vi "AlliGator Load mat FLI Dataset Information.vi"(8 "Error In":errorcluster, 9 "Laser Period":dbl[unit]=5.0000000000000004e-08, 11 "File Path":path) -> (0 "error out":errorcluster, 2 "Metadata":string, 3 "FLI Data File Information":T1, 4 "elapsed (relative) seconds":dbl)   [LabVIEW 2021, in "AlliGator Files.lvlib"]
doc: "Loads HDF5 FLI dataset information."
uses:
  AlliGator Files.lvlib
  HDF5/AlliGator FLI Data File Information.ctl
  Phasor/Phasor Fluorescence Lifetime Parameters v3.ctl
  AlliGator FLI Dataset Type.ctl
  AlliGator SS2 mat FLI File Loading Information.ctl
  AlliGator Load Single Gate Image from SS2 mat File.vi
  <vilib>/addons/h5labview2/base/lib_path.vi
  <vilib>/addons/h5labview2/base/H5Equery.vi
  <vilib>/addons/h5labview2/base/hid_t.ctl
  <vilib>/addons/h5labview2/dataset/H5Dread.llb/H5Dread.xnode
  <vilib>/addons/h5labview2/file/H5F.lvlib
  <vilib>/addons/h5labview2/group/H5G.lvlib
  Time/Time.lvlib
  HDF5/AlliGator HDF5.lvlib
  Phasor/Phasor.lvlib
panel:
  # "see the AlliGator License on the block diagram (Ctrl+E or Window:Show Block Diagram)"
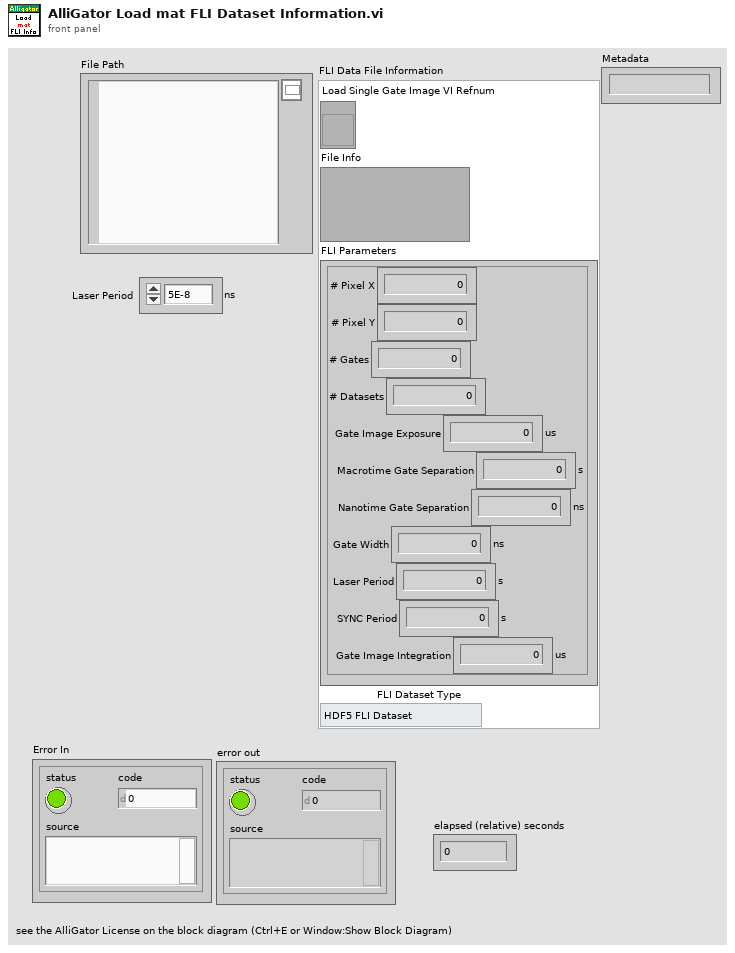
[diagram p1: front panel]
types:
  T1 = typedef "AlliGator HDF5.lvlib/AlliGator FLI Data File Information.ctl" = cluster{"Load Single Gate Image VI Refnum":refnum<vi>, "File Info":variant, "FLI Parameters":T2, "FLI Dataset Type":T3}
  T2 = typedef "Phasor.lvlib/Phasor Fluorescence Lifetime Parameters v3.ctl" = cluster{"# Pixel X":i32, "# Pixel Y":i32, "# Gates":i32, "# Datasets":i32, "Gate Image Exposure":dbl[unit], "Macrotime Gate Separation":dbl[unit], "Nanotime Gate Separation":dbl[unit], "Gate Width":dbl[unit], "Laser Period":dbl[unit], "SYNC Period":dbl[unit], "Gate Image Integration":dbl[unit]}
  T3 = typedef "AlliGator Files.lvlib/AlliGator FLI Dataset Type.ctl" = enum16{"HDF5 FLI Dataset", "Gate Image Folder", ".sdt FLI Dataset (Becker & Hickl)", ".ptu FLI Dataset (PicoQuant)", "SS1 FLI Dataset", "SS2 FLI Dataset", "I/m/phi Dataset", ".bin FLI Dataset (PicoQuant Binned)", ".bin FLI Dataset (Piccolo Binned)", ".mat FLI Dataset"}
  T4 = typedef "AlliGator Files.lvlib/AlliGator SS2 mat FLI File Loading Information.ctl" = cluster{"mat File Path":path, "# Datasets":i32, "# Gates/Dataset":i32}
  T5 = typedef "hid_t.ctl" = i64
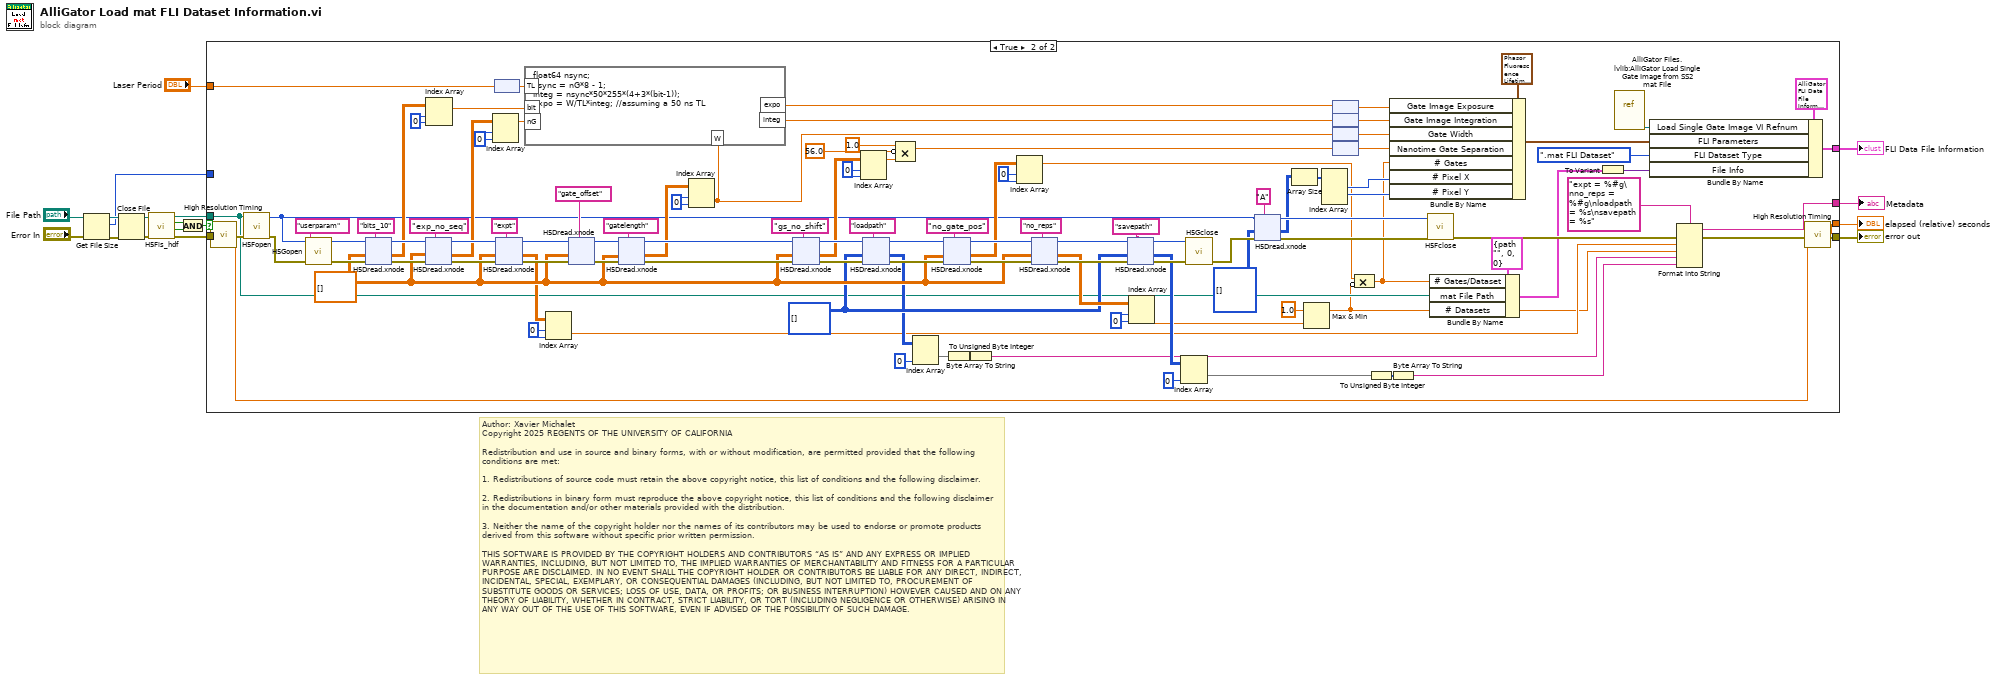
[diagram p0: block diagram]
diagram:
  # "Author: Xavier Michalet\nCopyright 2025 REGENTS OF THE UNIVERSITY OF CALIFORNIA\n\nRedistribution and use in source and binary forms, with or without modification, are permitted provided that the following conditions are met:\n\n1. Redistributions of source code must retain the above copyright notice, this list of conditions and the following disclaimer.\n\n2. Redistributions in binary form must reproduce the above copyright notice, this list of conditions and the following disclaimer in the documentation and/or other materials provided with the distribution.\n\n3. Neither the name of the copyright holder nor the names of its contributors may be used to endorse or promote products derived from this software without specific prior written permission.\n\nTHIS SOFTWARE IS PROVIDED BY THE COPYRIGHT HOLDERS AND CONTRIBUTORS “AS IS” AND ANY EXPRESS OR IMPLIED WARRANTIES, INCLUDING, BUT NOT LIMITED TO, THE IMPLIED WARRANTIES OF MERCHANTABILITY AND FITNESS FOR A PARTICULAR PURPOSE ARE DISCLAIMED. IN NO EVENT SHALL THE COPYRIGHT HOLDER OR CONTRIBUTORS BE LIABLE FOR ANY DIRECT, INDIRECT, INCIDENTAL, SPECIAL, EXEMPLARY, OR CONSEQUENTIAL DAMAGES (INCLUDING, BUT NOT LIMITED TO, PROCUREMENT OF SUBSTITUTE GOODS OR SERVICES; LOSS OF USE, DATA, OR PROFITS; OR BUSINESS INTERRUPTION) HOWEVER CAUSED AND ON ANY THEORY OF LIABILITY, WHETHER IN CONTRACT, STRICT LIABILITY, OR TORT (INCLUDING NEGLIGENCE OR OTHERWISE) ARISING IN ANY WAY OUT OF THE USE OF THIS SOFTWARE, EVEN IF ADVISED OF THE POSSIBILITY OF SUCH DAMAGE."
  n1 = Get File Size(file="File Path", error in="Error In") -> (refnum out=w8:refnum<file>, size (in bytes)=w3:i64, 0:w9:errorcluster)
  n2 = Close File(refnum=w8, error in=w9) -> (path=w7:path, error out=w6:errorcluster)
  n3 = call <vilib>:"H5Fis_hdf.vi"("error in (no error)"=w6, "path in"=w7) -> ("error out"=w13:errorcluster, "valid?"=w16:bool, "exists?"=w17:bool, "path out"=w14:path)  [unwired: 6 in]
  n4 = And(x=w17, y=w16) -> (x .and. y?=w15:bool)
  n5 = case shown="True" w15 {
    tunnel: w14 -> [_ w42]
    tunnel: w13 -> [w18 w128]
    tunnel: [w18 w126] -> w12
    tunnel: [_ w124] -> w5
    tunnel: [_ w116] -> w4
    tunnel: w3 -> [_ _]
    tunnel: "Laser Period" -> [_ w54]
    tunnel: [_ w34] -> w1
    frame False {
    }
    frame True {
      w58 = u16[][] []
      w59 = 0 ("disabled index (col)")
      w60 = 0 ("index (row)")
      w61 = 0 ("index (row)")
      w63 = 0 ("index (row)")
      w64 = 0 ("index (row)")
      w65 = 0 ("disabled index (col)")
      w67 = 0 ("index (row)")
      w85 = dbl[][] []
      n6 = call "High Resolution Timing.vi"("Error In"=w128) -> ("elapsed (relative) seconds"=w125:dbl, "Error Out"=w127:errorcluster)  [unwired: 16 in, 1 out]
      n7 = call <vilib>:"H5Fopen.vi"("error in (no error)"=w127, "path"=w42) -> ("error out"=w123:errorcluster, "ref out"=w33:T5)  [unwired: 8 in]
      n8 = call <vilib>:"H5Gopen.vi"("error in (no error)"=w123, "name"="userparam" ("dataset name (this)"), "ref in"=w33) -> ("error out"=w121:errorcluster, "group out"=w120:T5)  [unwired: 7 in]
      n9 = xnode "H5Dread.xnode"("dataset name (this)"="bits_10", "error in (no error)"=w121, "default"=w85, "ref in"=w120) -> ("error out"=w118:errorcluster, "data"=w74:dbl[][], "ref out"=w117:i64)  [unwired: 2 in, 1 out]
      n10 = xnode "H5Dread.xnode"("dataset name (this)"="exp_no_seq", "error in (no error)"=w118, "default"=w85, "ref in"=w117) -> ("error out"=w109:errorcluster, "data"=w75:dbl[][], "ref out"=w108:T5)  [unwired: 2 in, 1 out]
      n11 = Index Array(array=w74, index (row)=w67, index (col)=w67) -> (element=w68:dbl)
      n12 = Index Array(array=w75, index (row)=w65, index (col)=w65) -> (element=w66:dbl)
      n13 = node(w54) -> (w53:dbl)
      n14 = xnode "H5Dread.xnode"("dataset name (this)"="expt", "error in (no error)"=w109, "default"=w85, "ref in"=w108) -> ("error out"=w98:errorcluster, "data"=w70:dbl[][], "ref out"=w107:T5)  [unwired: 2 in, 1 out]
      n15 = Index Array(array=w70, index (row)=w64, index (col)=w64) -> (element=w37:dbl)
      n16 = xnode "H5Dread.xnode"("dataset name (this)"="gate_offset", "error in (no error)"=w98, "default"=w85, "ref in"=w107) -> ("error out"=w97:errorcluster, "ref out"=w106:T5)  [unwired: 2 in, 2 out]
      n17 = xnode "H5Dread.xnode"("dataset name (this)"="gatelength", "error in (no error)"=w97, "default"=w85, "ref in"=w106) -> ("error out"=w96:errorcluster, "data"=w83:dbl[][], "ref out"=w105:T5)  [unwired: 2 in, 1 out]
      n18 = Index Array(array=w83, index (row)=w63, index (col)=w63) -> (element=w57:dbl)
      n19 = formula code="float64 nsync;\nnsync = nG*8 - 1;\ninteg = nsync*50*255*(4+3*(bit-1));\nexpo = W/TL*integ; //assuming a 50 ns TL"("bit"=w68, "nG"=w66, "W"=w57, "TL"=w53) -> ("integ"=w73:dbl, "expo"=w55:dbl)
      n20 = xnode "H5Dread.xnode"("dataset name (this)"="gs_no_shift", "error in (no error)"=w96, "default"=w85, "ref in"=w105) -> ("error out"=w95:errorcluster, "data"=w80:dbl[][], "ref out"=w104:T5)  [unwired: 2 in, 1 out]
      n21 = Index Array(array=w80, index (row)=w61, index (col)=w61) -> (element=w62:dbl)
      n22 = xnode "H5Dread.xnode"("dataset name (this)"="loadpath", "error in (no error)"=w95, "default"=w58, "ref in"=w104) -> ("error out"=w94:errorcluster, "data"=w52:u16[][], "ref out"=w103:i64)  [unwired: 2 in, 1 out]
      n23 = Compound Arithmetic op=MULTIPLY(1.0 ("value"), invert 56.0 ("value"), w62) -> (w77:dbl)
      n24 = Index Array(array=w52, index (col)=0 ("disabled index (col)")) -> (element=w51:u16[])  [unwired: 1 in]
      n25 = xnode "H5Dread.xnode"("dataset name (this)"="no_gate_pos", "error in (no error)"=w94, "default"=w85, "ref in"=w103) -> ("error out"=w93:errorcluster, "data"=w81:dbl[][], "ref out"=w102:T5)  [unwired: 2 in, 1 out]
      n26 = To Unsigned Byte Integer(number=w51) -> (unsigned 8bit integer=w50:u8[])
      n27 = Byte Array To String(unsigned byte array=w50) -> (string=w36:string)
      n28 = Index Array(array=w81, index (row)=w60, index (col)=w60) -> (element=w20:dbl)
      n29 = xnode "H5Dread.xnode"("dataset name (this)"="no_reps", "error in (no error)"=w93, "default"=w85, "ref in"=w102) -> ("error out"=w92:errorcluster, "data"=w69:dbl[][], "ref out"=w101:T5)  [unwired: 2 in, 1 out]
      n30 = xnode "H5Dread.xnode"("dataset name (this)"="savepath", "error in (no error)"=w92, "default"=w58, "ref in"=w101) -> ("error out"=w99:errorcluster, "data"=w47:u16[][], "ref out"=w100:i64)  [unwired: 2 in, 1 out]
      n31 = Index Array(array=w69, index (row)=w59, index (col)=w59) -> (element=w23:dbl)
      n32 = Index Array(array=w47, index (col)=0 ("disabled index (col)")) -> (element=w48:u16[])  [unwired: 1 in]
      n33 = call <vilib>:"H5Gclose.vi"("error in (no error)"=w99, "group in"=w100) -> ("error out"=w32:errorcluster)  [unwired: 9 in]
      n34 = xnode "H5Dread.xnode"("dataset name (this)"="A", "error in (no error)"=w32, "default"=u16[][][] [], "ref in"=w33) -> ("error out"=w31:errorcluster, "data"=w28:u16[][][], "ref out"=w29:i64)  [unwired: 2 in, 1 out]
      n35 = Array Size(array=w28) -> (size(s)=w27:i32[])
      n36 = Max & Min(x=1.0, y=w23) -> (max(x,y)=w21:dbl)  [unwired: 1 out]
      n37 = Index Array(array=w27) -> (element #1=w26:i32, element #2=w25:i32)  [unwired: 3 in, 1 out]
      n38 = node(w55) -> (w56:dbl[unit])
      n39 = node(w73) -> (w72:dbl[unit])
      n40 = node(w57) -> (w82:dbl[unit])
      n41 = node(w77) -> (w76:dbl[unit])
      n42 = Compound Arithmetic op=MULTIPLY(w20, invert w21) -> (w19:dbl)
      n43 = To Unsigned Byte Integer(number=w48) -> (unsigned 8bit integer=w49:u8[])
      n44 = Bundle By Name(cluster=T2 {"# Pixel X"=0, "# Pixel Y"=0, "# Gates"=0, "# Datasets"=0, "Gate Image Exposure"=0.0, "Macrotime Gate Separation"=0.0, "Nanotime Gate Separation"=0.0, "Gate Width"=0.0, "Laser Period"=0.0, "SYNC Period"=0.0, "Gate Image Integration"=0.0} ("Swiss SPAD File Information"), "Gate Image Exposure"=w56, "Gate Image Integration"=w72, "Gate Width"=w82, "Nanotime Gate Separation"=w76, "# Gates"=w19, "# Pixel X"=w26, "# Pixel Y"=w25) -> (w71:T2)
      n45 = Byte Array To String(unsigned byte array=w49) -> (string=w35:string)
      n46 = call <vilib>:"H5Fclose.vi"("error in (no error)"=w31, "ref"=w29) -> ("error out"=w87:errorcluster)  [unwired: 9 in]
      n47 = Bundle By Name(cluster=T4 {"mat File Path"=path "", "# Datasets"=0, "# Gates/Dataset"=0} ("SS2 mat File Loading Information"), "# Gates/Dataset"=w19, "mat File Path"=w42, "# Datasets"=w21) -> (w41:T4)
      n48 = To Variant(anything=w41) -> (Variant=w40:variant)
      n49 = vi-ref "AlliGator Files.lvlib:AlliGator Load Single Gate Image from SS2 mat File.vi"() -> (w114:refnum<vi>)
      n50 = Bundle By Name(cluster=T1 {"Load Single Gate Image VI Refnum"=refnum, "File Info"=variant, "FLI Parameters"={"# Pixel X"=0, "# Pixel Y"=0, "# Gates"=0, "# Datasets"=0, "Gate Image Exposure"=0.0, "Macrotime Gate Separation"=0.0, "Nanotime Gate Separation"=0.0, "Gate Width"=0.0, "Laser Period"=0.0, "SYNC Period"=0.0, "Gate Image Integration"=0.0}, "FLI Dataset Type"=enum."HDF5 FLI Dataset"} ("FLI Data File Information"), "Load Single Gate Image VI Refnum"=w114, "FLI Parameters"=w71, "FLI Dataset Type"=AlliGator_FLI_Dataset_Type.".mat FLI Dataset", "File Info"=w40) -> (w116:T1)
      n51 = Format Into String(format string="expt = %#g\nno_reps = %#g\nloadpath = %s\nsavepath = %s", error in=w87, w37, w21, w36, w35) -> (resulting string=w34:string, error out=w39:errorcluster)  [unwired: 1 in]
      n52 = call "High Resolution Timing.vi"("relative seconds (NaN)"=w125, "Error In"=w39) -> ("elapsed (relative) seconds"=w124:dbl, "Error Out"=w126:errorcluster)  [unwired: 15 in, 1 out]
    }
  }
  "error out" <- w12
  "elapsed (relative) seconds" <- w5
  "FLI Data File Information" <- w4
  "Metadata" <- w1
